vi "读取高速数据(M).vi"(8 "错误输入":errorcluster caption="错误输入（无错误）", 10 "数据个数":i32, 11 "设备句柄入":i32) -> (0 "错误输出":errorcluster, 1 "返回数据个数":i32, 2 "原码值":u16[](array[numeric]), 3 "设备句柄":i32=1)   [LabVIEW 2016]
uses:
  dll/em9636.dll
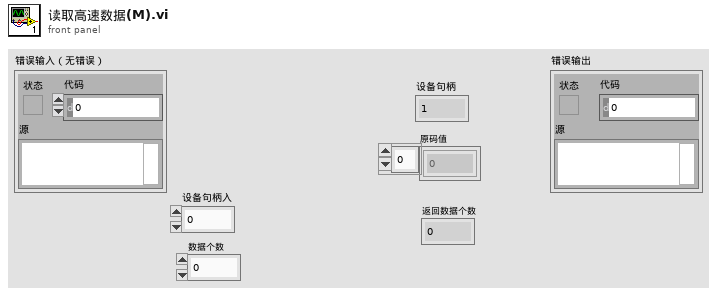
[diagram p1: front panel]
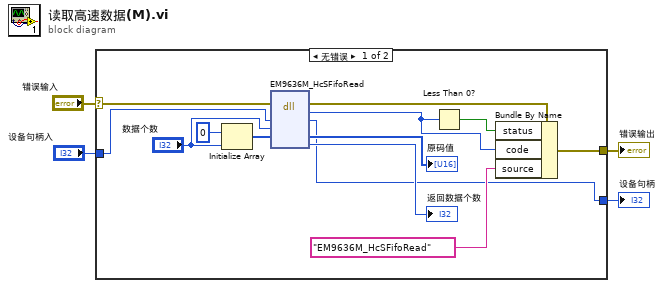
[diagram p0: block diagram]
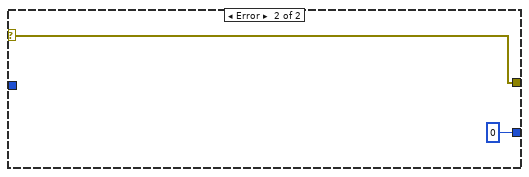
[diagram p2: hidden frame]
diagram:
  n1 = case shown="无错误" "错误输入" {
    selector: "错误输入" -> [w17 w19]
    tunnel: [w13 w19] -> w3
    tunnel: [w5 0 ("错误")] -> w2
    tunnel: "设备句柄入" -> [w11 _]
    frame No Error {
      n2 = Initialize Array(u16 0 ("元素"), "数据个数") -> (w7:u16[])
      n3 = dll-call lib="PTH2kabs CUsers\nAdministratorDesktopEM9636*EM9636系列_demo_labview(调用DLL方式)dll\nem9636.dll" fn="EM9636M_HcSFifoRead"(error in=w17, "设备句柄"=w11, "数据个数"="数据个数", "原码值"=w7) -> (error out=w15:errorcluster, "错误"=w12:i32, "设备句柄"=w5:i32, "原码值"=→"原码值":u16[], "返回数据个数"=→"返回数据个数":i32)  [unwired: 4 in, 1 out]
      n4 = Less Than 0?(x=w12) -> (x < 0?=w14:bool)
      n5 = Bundle By Name(cluster=w15, "status"=w14, "code"=w12, "source"="EM9636M_HcSFifoRead") -> (w13:errorcluster)
    }
    frame Error {
    }
  }
  "错误输出" <- w3
  "设备句柄" <- w2
